vi "SIM921_merge_cluster.vi"(0 "SIM921-Status":T2, 1 "SIM921-Control":T3) -> (3 "SIM921":T1)   [LabVIEW 2019]
uses:
  SIM921/SIM921_control_cluster.ctl
  SIM921/SIM921_status_cluster.ctl
  SIM921/SIM921_resistance_Bridge_cluster.ctl
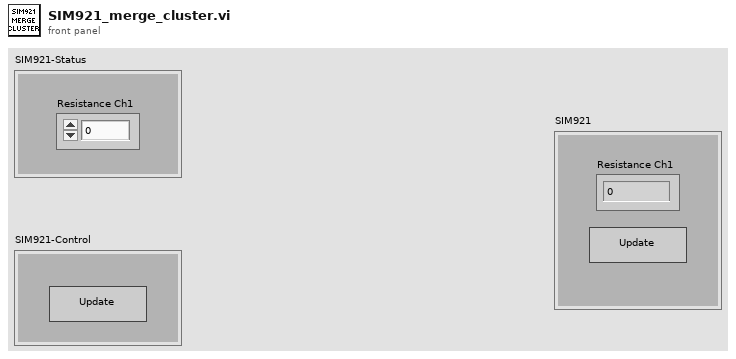
[diagram p1: front panel]
types:
  T1 = typedef "SIM921_resistance_Bridge_cluster.ctl" = cluster{"Resistance Ch1":dbl, "Update":bool}
  T2 = typedef "SIM921_status_cluster.ctl" = cluster{"Resistance Ch1":dbl}
  T3 = typedef "SIM921_control_cluster.ctl" = cluster{"Update":bool}
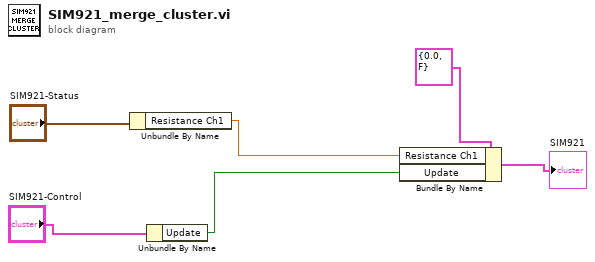
[diagram p0: block diagram]
diagram:
  n1 = Unbundle By Name("SIM921-Status") -> ("Resistance Ch1"=w2:dbl)
  n2 = Unbundle By Name("SIM921-Control") -> ("Update"=w1:bool)
  n3 = Bundle By Name(cluster=T1 {"Resistance Ch1"=0.0, "Update"=FALSE} ("SIM921"), "Resistance Ch1"=w2, "Update"=w1) -> (→"SIM921":T1)
